vi "Export scale.vi"(5 "Folder":T1=enum."PublicAppFolder", 7 "error in (no error)":errorcluster, 10 "Index":u32) -> (0 "error":errorcluster)   [LabVIEW 2015]
uses:
  Process Controller 3.0/Calibration and Function folders.ctl
  DAQ configuration/Sensor buffer command.ctl
panel:
  out "Array":dbl[][](array[numeric])
  out "Photometer data in.Standards":cluster{"Concentration":dbl, "Voltage":dbl}[](array[cluster])
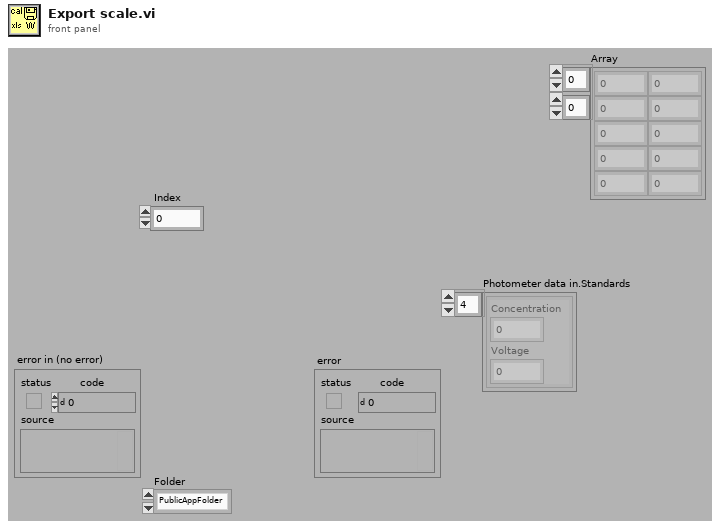
[diagram p1: front panel]
types:
  T1 = typedef "Calibration and Function folders.ctl" = enum16{"Sensors", "Functions", "Config File", "PublicAppFolder", "New ini File", "Set Config File", "Delete ini File"}
  T2 = typedef "Sensor buffer command.ctl" = enum16{"read average", "read recent", "read all", "write", "set buffer size", "Read channel config", "Write channel config", "clear"}
  T3 = enum16{"open", "open or create", "create or replace", "create", "open (read only)"}
  T4 = typedef "Channel config.ctl" = cluster{"Channel Indices":T5[], "AI Max voltage":dbl[], "Calibration matrix":T6}
  T5 = typedef "channel identifier.ctl" = u16
  T6 = typedef "calib array.ctl" = T7[]
  T7 = typedef "conversion.ctl" = cluster{"conversion matrix":sgl[][], "units":string, "name":string, "scale type":T8, "offset (volts)":dbl, "second channel":i8, "correspondence table":T9, "offset (physical units)":dbl, "pH scale":T10, "D.O.":T11, "Photometer data":T12}
  T8 = typedef "scale type.ctl" = enum16{"Volts", "Polynomial", "Correspondence Table", "pH", "Dissolved Oxygen", "Quadratic", "Photometer"}
  T9 = typedef "correspondence table.ctl" = cluster{"physical units":dbl, "volts":dbl}[]
  T10 = typedef "pH scale.ctl" = cluster{"Buffers":cluster{"Buffer":dbl, "Calibrated":bool, "V/T":dbl}[], "Temperature":dbl}
  T11 = typedef "DO scale.ctl" = cluster{"Temperature":dbl, "K":dbl, "barometric pressure":dbl}
  T12 = typedef "Photometer calibration data.ctl" = cluster{"Dark Voltage":dbl, "Blank Voltage":dbl, "Standards":cluster{"Concentration":dbl, "Voltage":dbl}[]}
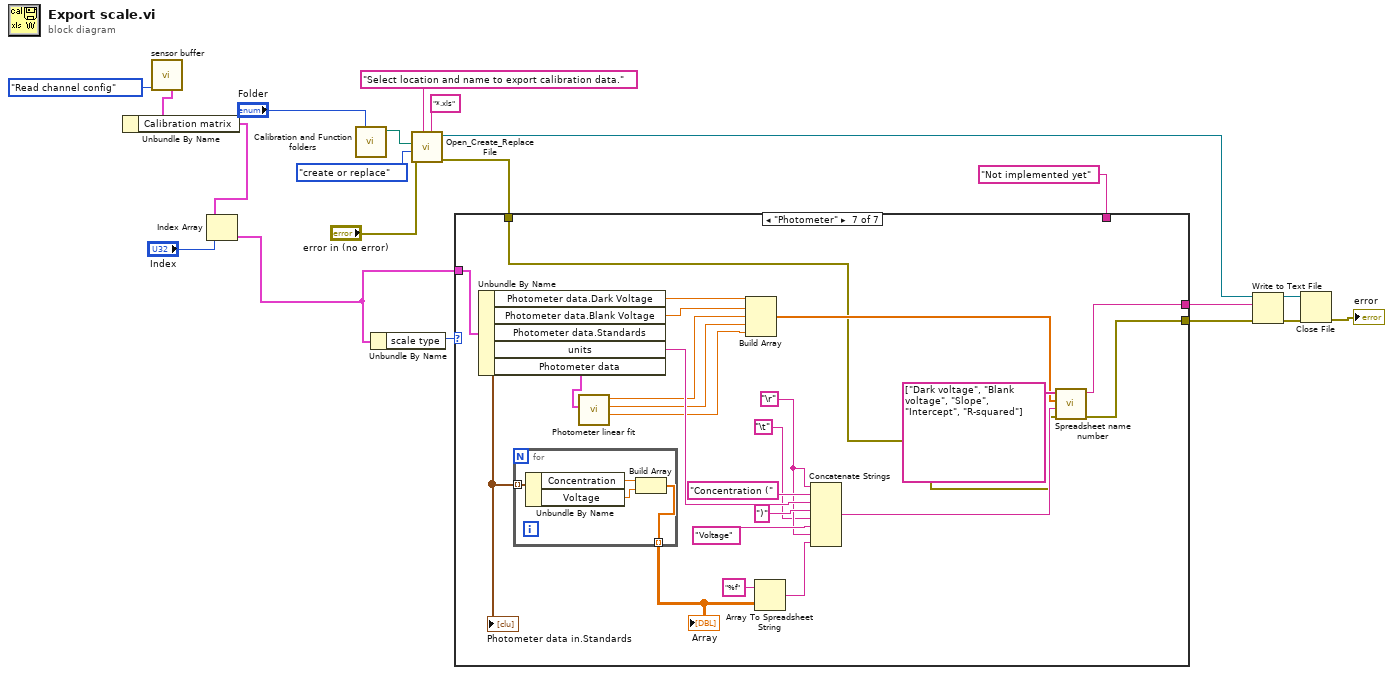
[diagram p0: block diagram]
diagram:
  n1 = call "sensor buffer.vi"("command"=Sensor_buffer_command."Read channel config") -> ("Channel Config out"=w15:T4)  [unwired: 6 in, 4 out]
  n2 = Unbundle By Name(w15) -> ("Calibration matrix"=w14:T6)
  n3 = Index Array(array=w14, index="Index") -> (element=w9:T7)
  n4 = call "Calibration and Function folders.vi"("Folder"="Folder") -> ("Selected Folder"=w13:path)  [unwired: 9 in, 1 out]
  n5 = Unbundle By Name(w9) -> ("scale type"=w10:T8)
  n6 = call <vilib>:"Open_Create_Replace File.vi"("pattern"="*.xls", "prompt"="Select location and name to export calibration data.", "error in (no error)"="error in (no error)", "function (open:0)"=T3."create or replace", "start path  (Not A Path)"=w13) -> ("error out"=w6:errorcluster, "refnum"=w7:refnum<file>)  [unwired: 3 in, 2 out]
  n7 = case shown="\"Photometer\"" w10 {
    tunnel: w9 -> [_ _ _ _ _ _ w47]
    tunnel: [w22 w24 w26 w28 w30 w32 w35] -> w8
    tunnel: w6 -> [w21 w23 w25 w27 w29 w31 w33]
    tunnel: [w21 w23 w25 w27 w29 w31 w34] -> w5
    tunnel: "Not implemented yet" -> [w22 w24 w26 w28 w30 w32 _]
    frame "Volts", Default {
    }
    frame "Polynomial" {
    }
    frame "Correspondence Table" {
    }
    frame "pH" {
    }
    frame "Dissolved Oxygen" {
    }
    frame "Quadratic" {
    }
    frame "Photometer" {
      w44 = "\r"
      n8 = Unbundle By Name(w47) -> ("Photometer data.Dark Voltage"=w42:dbl, "Photometer data.Blank Voltage"=w41:dbl, "Photometer data.Standards"=w55:cluster{"Concentration":dbl, "Voltage":dbl}[], "units"=w53:string, "Photometer data"=w46:T12)
      "Photometer data in.Standards" <- w55
      n9 = for {
        tunnel: w55 -> [w59] mode=indexing
        tunnel: [w56] -> w50 mode=indexing
        n10 = Unbundle By Name(w59) -> ("Concentration"=w58:dbl, "Voltage"=w57:dbl)
        n11 = Build Array(w58, w57) -> (w56:dbl[])
      }
      "Array" <- w50
      n12 = call "Photometer linear fit.vi"("Photometer data in"=w46) -> ("R-square"=w38:dbl, "intercept"=w39:dbl, "slope"=w40:dbl)  [unwired: 7 in, 1 out]
      n13 = Build Array(w42, w41, w40, w39, w38) -> (w37:dbl[])
      n14 = Array To Spreadsheet String(array=w50, 3:"%f" ("format string")) -> (spreadsheet string=w49:string)  [unwired: 1 in]
      n15 = Concatenate Strings(w44, "Concentration (", w53, ")" ("string"), "\t", "Voltage", w44, w49) -> (w36:string)
      n16 = call "Spreadsheet name number.vi"("error in"=w33, "Terminal String"=w36, "Numbers"=w37, "Names"=string[] ["Dark voltage", "Blank voltage", "Slope", "Intercept", "R-squared"]) -> ("error out"=w34:errorcluster, "Spreadsheet String"=w35:string)  [unwired: 6 in]
    }
  }
  n17 = Write to Text File(file (use dialog)=w7, text=w8, error in=w5) -> (refnum out=w3:refnum<file>, error out=w4:errorcluster)  [unwired: 1 in, 1 out]
  n18 = Close File(refnum=w3, error in=w4) -> (error out=→"error":errorcluster)  [unwired: 1 out]
